vi "Send Command.vi"(8 "error in (no error)":errorcluster, 10 "write buffer":string, 11 "VISA resource name":refnum<visa-resource-name>) -> (0 "error out":errorcluster, 3 "VISA resource name out":refnum<visa-resource-name>)   [LabVIEW 2012, in "Tektronix AFG 3000 Series.lvlib"]
doc: "Acquires a lock on the specified AFG3000 series function generator, sends the given command, and checks for errors."
uses:
  Tektronix AFG 3000 Series.lvlib
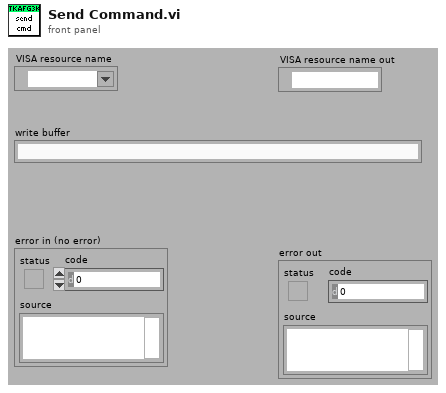
[diagram p1: front panel]
types:
  T1 = typedef "Semaphore RefNum" = refnum<k1>
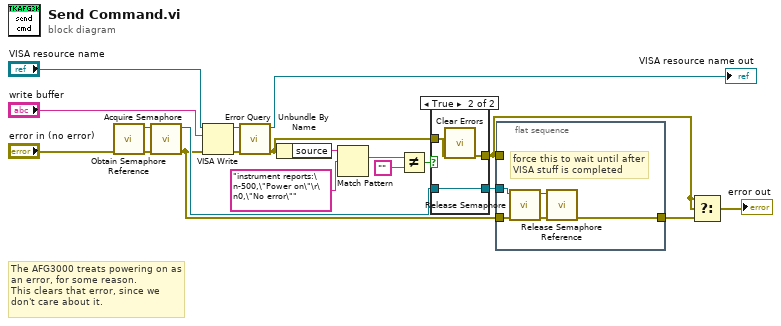
[diagram p0: block diagram]
diagram:
  # "The AFG3000 treats powering on as an error, for some reason.\nThis clears that error, since we don't care about it."
  n1 = call <vilib>:"Obtain Semaphore Reference.vi"("error in (no error)"="error in (no error)") -> ("error out"=w14:errorcluster, "semaphore"=w17:T1)  [unwired: 2 in, 3 out]
  n2 = call <vilib>:"Acquire Semaphore.vi"("error in (no error)"=w14, "semaphore"=w17) -> ("error out"=w2:errorcluster, "semaphore out"=w6:T1)  [unwired: 1 in, 3 out]
  n3 = VISA Write(VISA resource name="VISA resource name", write buffer="write buffer", error in (no error)=w2) -> (VISA resource name out=w19:refnum<visa-resource-name>, error out=w20:errorcluster)  [unwired: 1 out]
  n4 = call "Error Query.vi"("error in (no error)"=w20, "VISA resource name"=w19) -> ("error out"=w12:errorcluster, "VISA resource name out"=→"VISA resource name out":refnum<visa-resource-name>)  [unwired: 8 out]
  n5 = Unbundle By Name(w12) -> ("source"=w9:string)
  n6 = Match Pattern(string=w9, regular expression="instrument reports:\n-500,\"Power on\"\r\n0,\"No error\"") -> (match substring=w8:string)  [unwired: 4 out]
  n7 = Not Equal?(x=w8, y="") -> (x != y?=w7:bool)
  n8 = case shown="True" w7 {
    tunnel: w12 -> [w21 w25]
    tunnel: [w21 w24] -> w1
    tunnel: w6 -> [w22 w23]
    tunnel: [w22 w23] -> w5
    frame False {
    }
    frame True {
      n9 = call <vilib>:"Clear Errors.vi"("error in (no error)"=w25) -> ("error out"=w24:errorcluster)  [unwired: 6 out]
    }
  }
  n10 = flat-sequence {
    tunnel: [w29] -> w3
    tunnel: w2 -> [w27]
    tunnel: w5 -> [w26]
    tunnel: w1 -> [_]
    frame #0 {
      # "force this to wait until after \nVISA stuff is completed"
      n11 = call <vilib>:"Release Semaphore.vi"("error in (no error)"=w27, "semaphore"=w26) -> ("error out"=w30:errorcluster, "semaphore out"=w28:T1)  [unwired: 4 out]
      n12 = call <vilib>:"Release Semaphore Reference.vi"("error in (no error)"=w30, "semaphore"=w28) -> ("error out"=w29:errorcluster)  [unwired: 9 out]
    }
  }
  n13 = Select(t=w1, s=w1, f=w3) -> (s? t:f=→"error out":errorcluster)
